vi "Save DB Images.vi"(1 "Images to Keep":dbl=60.0, 2 "Time Interval (s)":dbl=1.0, 3 "Image":T1) -> ()   [LabVIEW 2011]
uses:
  <vilib>/vision/Image Controls.llb/IMAQ Image.ctl
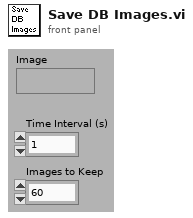
[diagram p1: front panel]
types:
  T1 = typedef "IMAQ Image.ctl" = refnum<image>
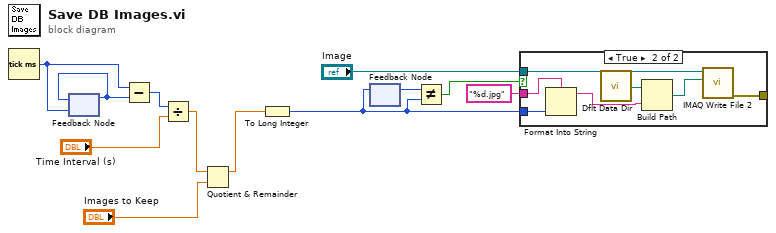
[diagram p0: block diagram]
diagram:
  n1 = Tick Count (ms)() -> (millisecond timer value=w11:u32)
  n2 = feedback #1(w11) -> (w10:u32)
  n3 = feedback-in #1(w10) -> ()
  n4 = Subtract(x=w11, y=w10) -> (x-y=w12:u32)
  n5 = Divide(x=w12, y="Time Interval (s)") -> (x/y=w7:dbl)
  n6 = Quotient & Remainder(x=w7, y="Images to Keep") -> (x-y*floor(x/y)=w6:dbl)  [unwired: 1 out]
  n7 = To Long Integer(number=w6) -> (32bit integer=w8:i32)
  n8 = feedback #2() -> (w3:i32)  [unwired: 1 out]
  n9 = feedback-in #2(w8) -> ()
  n10 = Not Equal?(x=w3, y=w8) -> (x != y?=w4:bool)
  n11 = case shown="True" w4 {
    tunnel: "Image" -> [_ w19]
    tunnel: [_ w16] -> _
    tunnel: "%d.jpg" ("format string") -> [_ w13]
    tunnel: w8 -> [_ w14]
    frame False {
    }
    frame True {
      n12 = Format Into String(format string=w13, w14) -> (resulting string=w15:string)  [unwired: 2 in, 1 out]
      n13 = call <vilib>:"Dflt Data Dir.vi"() -> ("App:Default Data Directory"=w18:path)
      n14 = Build Path(base path=w18, name or relative path=w15) -> (appended path=w17:path)
      n15 = call-poly "IMAQ Write File 2"("File Path"=w17, "Image"=w19) -> ("error out"=w16:errorcluster)  [unwired: 3 in, 6 out]
    }
  }
